vi "Create and Read CDO.vi"(8 "error in":errorcluster, 9 "drive from slot in":T1, 10 "channel settings in":T2[](array[typedef]), 11 "NI 9474 test in":refnum<class "NI 9474 Test.lvclass">) -> (0 "error out":errorcluster, 1 "drive from slot out":T1, 2 "channel settings out":T2[](array[typedef]), 3 "NI 9474 test out":refnum<class "NI 9474 Test.lvclass">)   [LabVIEW 2020, in "NI 9474 Test.lvclass"]
uses:
  NI 9474 Test.lvclass
  Scripting/Modules/Mode Classes/Controls/counter driven output channel settings.ctl
  Scripting/Modules/Channel Classes/Counter Driven Output Channel/Counter Driven State.ctl
  Scripting/Modules/Mode Classes/Counter Driven Output Mode/Drive from Slot.ctl
  Scripting/Modules/NI 9474/NI 9474.lvclass
  Scripting/Modules/Channel Classes/Counter Driven Output Channel/Counter Driven Output Channel.lvclass
  Scripting/Scan Engine Scripting.lvlib
  Scripting/Modules/Mode Classes/Counter Driven Output Mode/Counter Driven Output Mode.lvclass
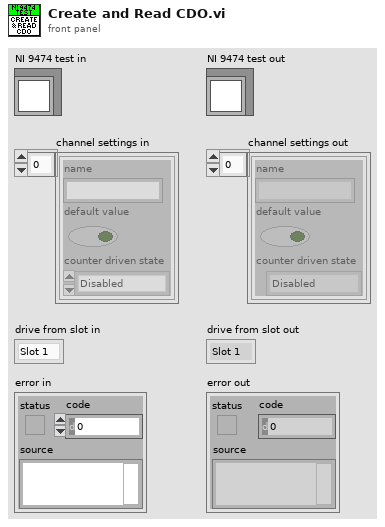
[diagram p1: front panel]
types:
  T1 = typedef "Scan Engine Scripting.lvlib/Counter Driven Output Mode.lvclass/Drive from Slot.ctl" = enum16{"Slot 1", "Slot 2", "Slot 3", "Slot 4", "Slot 5", "Slot 6", "Slot 7", "Slot 8"}
  T2 = typedef "Scan Engine Scripting.lvlib/counter driven output channel settings.ctl" = cluster{"name":string, "default value":bool, "counter driven state":T3}
  T3 = typedef "Scan Engine Scripting.lvlib/Counter Driven Output Channel.lvclass/Counter Driven State.ctl" = enum16{"Disabled", "Enabled"}
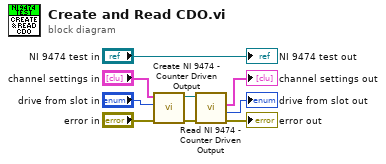
[diagram p0: block diagram]
diagram:
  n1 = call "Create NI 9474 - Counter Driven Output.vi"("error in"="error in", "drive from slot"="drive from slot in", "channel settings"="channel settings in") -> ("error out"=w9:errorcluster, "NI 9474 out"=w7:refnum<class "NI 9474.lvclass">)  [unwired: 7 in]
  n2 = call "Read NI 9474 - Counter Driven Output.vi"("error in"=w9, "NI 9474 in"=w7) -> ("error out"=→"error out":errorcluster, "drive from slot"=→"drive from slot out":T1, "channel settings"=→"channel settings out":T2[])  [unwired: 6 in, 1 out]
  "NI 9474 test out" <- "NI 9474 test in"
